vi "Fit.vi"(7 "Type X":T1(ring), 8 "error in (no error)":errorcluster caption="entrée d'erreur (pas d'erreur)", 10 "X":string[][](array[string]), 11 "MissingIndicator.lvclass":refnum<class "MissingIndicator.lvclass">) -> (0 "error out":errorcluster caption="sortie d'erreur", 2 "String Data":string, 3 "MissingIndicator.lvclass":refnum<class "MissingIndicator.lvclass">)   [LabVIEW 2020, in "MissingIndicator.lvclass"]
doc: "Fit the transformer on X.\n\nReturns : \n\n- String : OK"
uses:
  MissingIndicator.lvclass
  MissingIndicator.lvclass/MissingIndicator.ctl
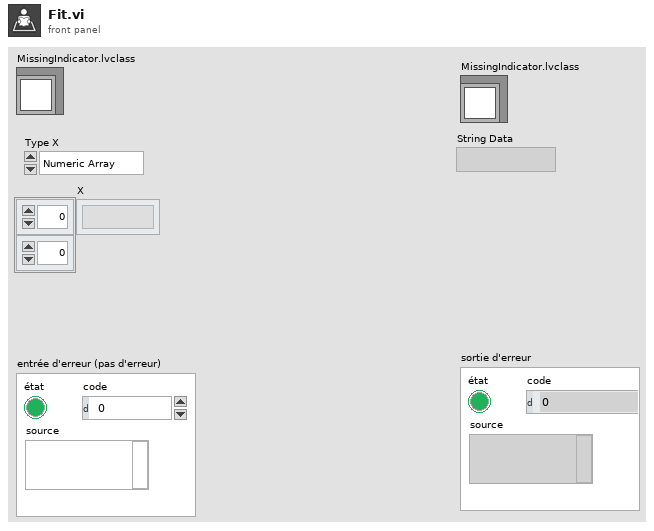
[diagram p1: front panel]
types:
  T1 = enum16{"Numeric Array", "String Array", "Sparse"}
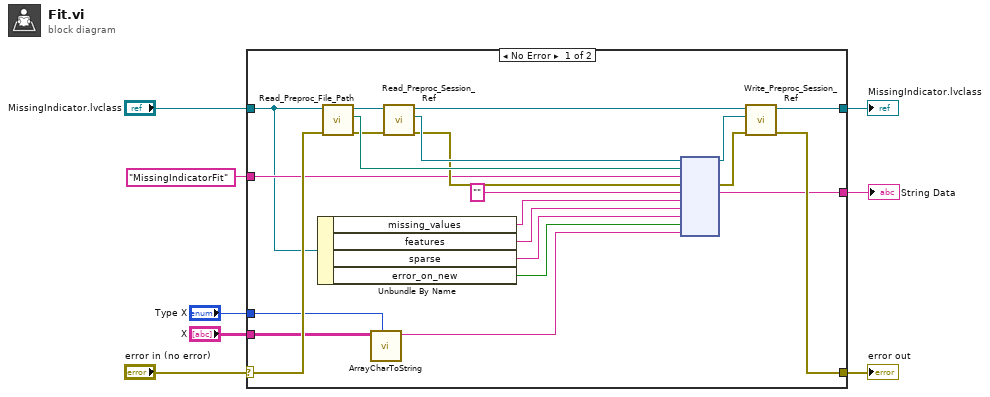
[diagram p0: block diagram]
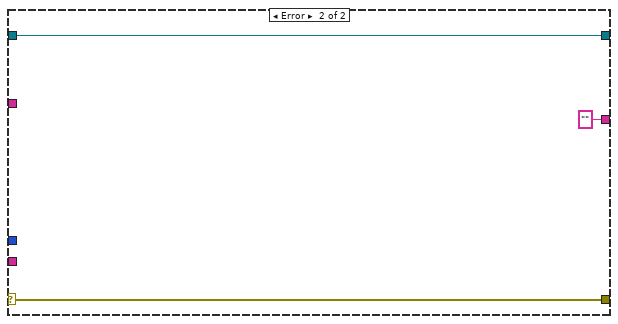
[diagram p2: hidden frame]
diagram:
  n1 = case shown="No Error" "error in (no error)" {
    selector: "error in (no error)" -> [w21 w33]
    tunnel: [w20 w33] -> w7
    tunnel: [w19 w32] -> w5
    tunnel: "MissingIndicator.lvclass" -> [w16 w32]
    tunnel: "MissingIndicatorFit" ("Fonction") -> [w18 _]
    tunnel: [w17 ""] -> w3
    tunnel: "X" -> [w11 _]
    tunnel: "Type X" -> [w9 _]
    frame No Error {
      n2 = Unbundle By Name(w16) -> ("missing_values"=w15:string, "features"=w14:string, "sparse"=w13:string, "error_on_new"=w12:bool)
      n3 = call-dynamic "Read_Preproc_File_Path.vi"("error in (no error)"=w21, "Python in"=w16) -> ("error out"=w25:errorcluster, "File_Path"=w28:path, "Python out"=w30:refnum<class "MissingIndicator.lvclass">)  [unwired: 7 in]
      n4 = call "ArrayCharToString.vi"("Type"=w9, "TAB"=w11) -> ("Instruction"=w10:string)  [unwired: 9 in]
      n5 = call-dynamic "Read_Preproc_Session_Ref.vi"("error in (no error)"=w25, "Python in"=w30) -> ("error out"=w26:errorcluster, "Session_ref"=w27:refnum<k35>, "Python out"=w29:refnum<class "MissingIndicator.lvclass">)  [unwired: 7 in]
      n6 = node(w27, w28, w18, w26, "", w15, w14, w13, w12, w10) -> (w22:refnum<k35>, w24:errorcluster, w17:string)  [unwired: 5 in, 2 out]
      n7 = call-dynamic "Write_Preproc_Session_Ref.vi"("error in (no error)"=w24, "Session_ref"=w22, "Python in"=w29) -> ("error out"=w20:errorcluster, "Python out"=w19:refnum<class "MissingIndicator.lvclass">)  [unwired: 7 in]
    }
    frame Error {
    }
  }
  "error out" <- w7
  "MissingIndicator.lvclass" <- w5
  "String Data" <- w3
